vi "MDAQ_WriteFileHeader.vi"(7 "Sample Name":string, 8 "error in":errorcluster, 9 "Control Cluster":T1 {"CV"."Temperature Array" scale=0.0..100.0}, 10 "User Comment":string, 11 "FileRef In":refnum<file>) -> (0 "error out":errorcluster, 1 "Control Cluster Out":T1 {"CV"."Temperature Array" scale=0.0..100.0}, 3 "refnum out":refnum<file>)   [LabVIEW 2021]
uses:
  GUI_Def.ctl
  Mode_Enum.ctl
  XML_Cluster.ctl
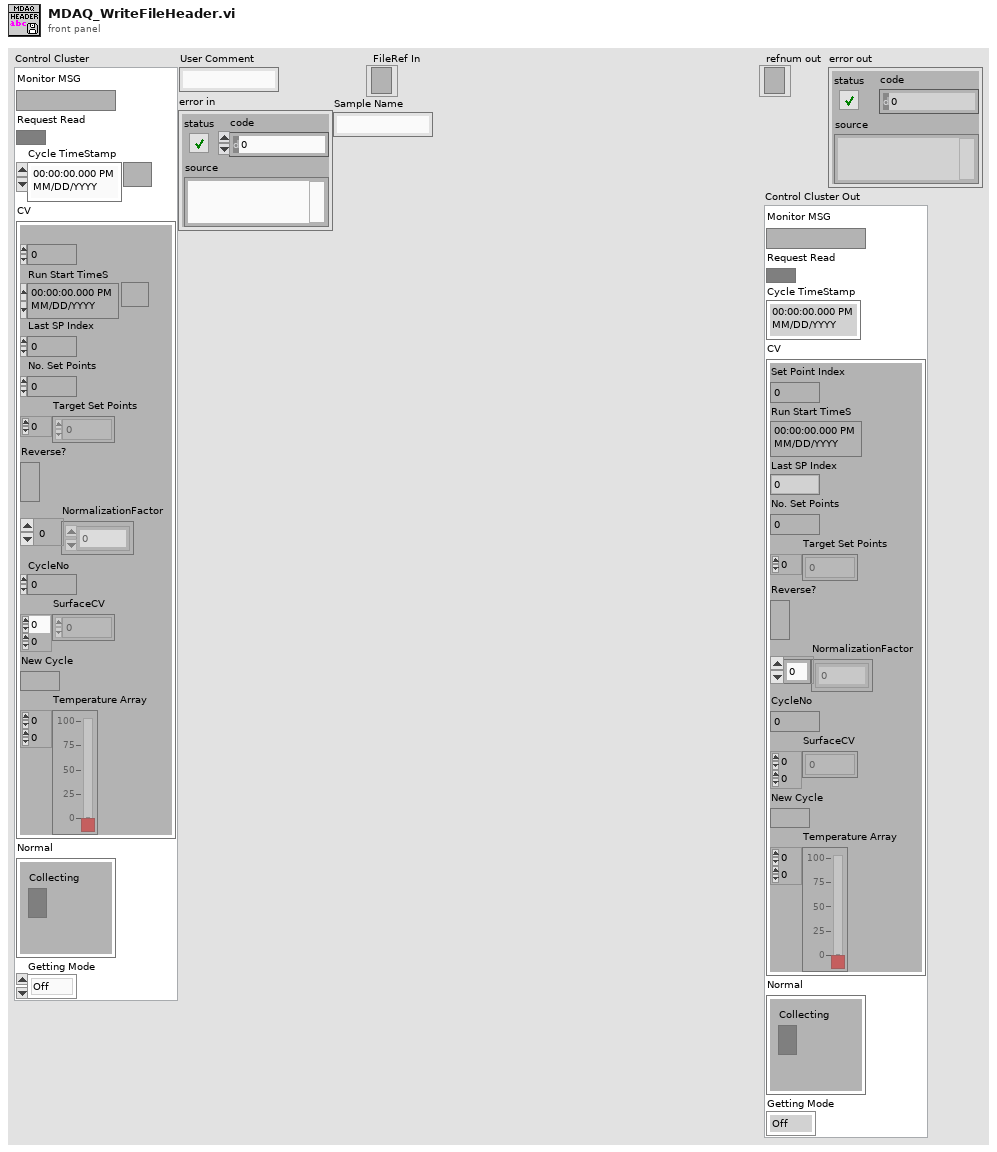
[diagram p1: front panel]
types:
  T1 = typedef "GUI_Def.ctl" = cluster{"Monitor MSG":string, "Request Read":bool, "Cycle TimeStamp":timestamp, "CV":cluster{"Set Point Index":u32, "Run Start TimeS":timestamp, "Last SP Index":u32, "No. Set Points":u32, "Target Set Points":i32[], "Reverse?":bool, "NormalizationFactor":i32[], "CycleNo":i32, "SurfaceCV":dbl[][], "New Cycle":bool, "Temperature Array":dbl[][]}, "Normal":cluster{"Collecting":bool}, "Getting Mode":T2}
  T2 = typedef "Mode_Enum.ctl" = enum16{"Off", "Normal", "CV+Temp", "CV"}
  T3 = typedef "XML_Cluster.ctl" = cluster{"User Comment":string, "Run Start TimeS":timestamp, "No. Set Points":u32, "Target Set Points":i32[], "Sample Name":string}
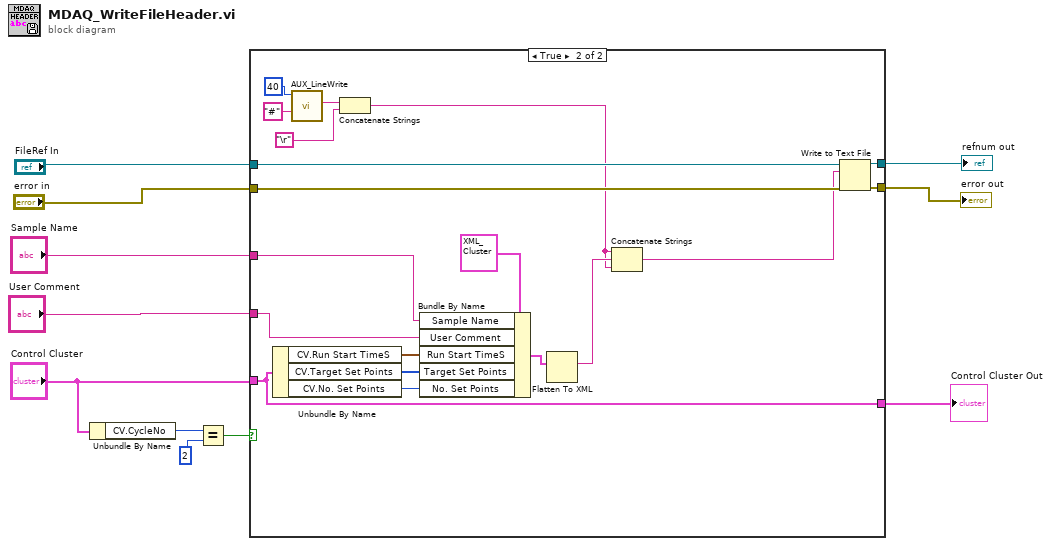
[diagram p0: block diagram]
diagram:
  n1 = Unbundle By Name("Control Cluster") -> ("CV.CycleNo"=w10:i32)
  n2 = Equal?(x=w10, y=2) -> (x = y?=w8:bool)
  n3 = case shown="True" w8 {
    tunnel: "Control Cluster" -> [w12 w17]
    tunnel: "FileRef In" -> [w14 w33]
    tunnel: "User Comment" -> [_ w28]
    tunnel: "error in" -> [w13 w32]
    tunnel: [w14 w20] -> w4
    tunnel: [w13 w19] -> w3
    tunnel: "Sample Name" -> [_ w18]
    tunnel: [w12 w17] -> w1
    frame False {
    }
    frame True {
      n4 = Unbundle By Name(w17) -> ("CV.Run Start TimeS"=w27:timestamp, "CV.Target Set Points"=w26:i32[], "CV.No. Set Points"=w25:u32)
      n5 = call "AUX_LineWrite.vi"("String"="#", "Char Number"=40) -> ("Line Out"=w30:string)  [unwired: 9 in]
      n6 = Concatenate Strings(w30, "\r") -> (w16:string)
      n7 = Bundle By Name(cluster=T3 {"User Comment"="", "Run Start TimeS"=timestamp(0 s since 1904-01-01), "No. Set Points"=0, "Target Set Points"=[], "Sample Name"=""} ("Cluster"), "Sample Name"=w18, "User Comment"=w28, "Run Start TimeS"=w27, "Target Set Points"=w26, "No. Set Points"=w25) -> (w23:T3)
      n8 = Flatten To XML(6:w23) -> (2:w22:string)
      n9 = Concatenate Strings(w16, w22, w16) -> (w21:string)
      n10 = Write to Text File(file (use dialog)=w33, text=w21, error in=w32) -> (refnum out=w20:refnum<file>, error out=w19:errorcluster)  [unwired: 1 in, 1 out]
    }
  }
  "refnum out" <- w4
  "error out" <- w3
  "Control Cluster Out" <- w1
